vi "UpgradeVIPBVersion.vi"(11 "CommandLineIn":string[](array[string])) -> (2 "output":string, 3 "return code":i32)   [LabVIEW 2019]
panel:
  in  "error in":errorcluster
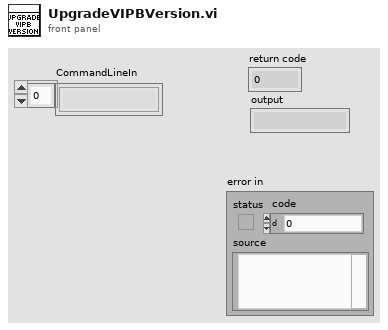
[diagram p1: front panel]
types:
  T1 = typedef "VIPM API_vipm_api.lvlib/Version Info Cluster_vipm_api.ctl" = cluster{"major":u32, "minor":u32, "patch":u32, "build":u32}
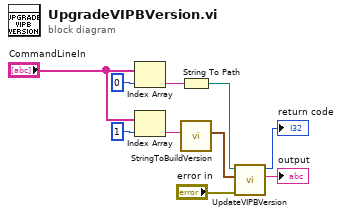
[diagram p0: block diagram]
diagram:
  n1 = Index Array(array="CommandLineIn", index=0) -> (element=w6:string)
  n2 = Index Array(array="CommandLineIn", index=1) -> (element=w7:string)
  n3 = String To Path(string=w6) -> (path=w5:path)
  n4 = call "StringToBuildVersion.vi"("Version string"=w7) -> ("Version"=w4:T1)  [unwired: 10 in]
  n5 = call "UpdateVIPBVersion.vi"("error in (no error)"="error in", "Updated Package Version"=w4, "Path to VIPB File"=w5) -> ("output"=→"output":string, "return code"=→"return code":i32)  [unwired: 7 in]
